vi "get_output_type.vi"(8 "error in (no error)":errorcluster, 11 "VISA Refnum in":refnum<visa-resource-name>) -> (0 "error out":errorcluster, 2 "Output type":string, 3 "VISA Refnum out":refnum<visa-resource-name>)   [LabVIEW 2018]
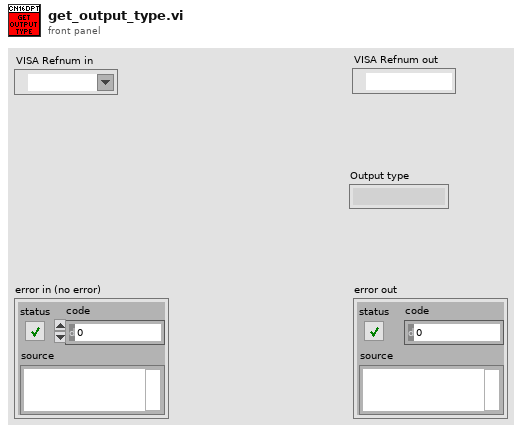
[diagram p1: front panel]
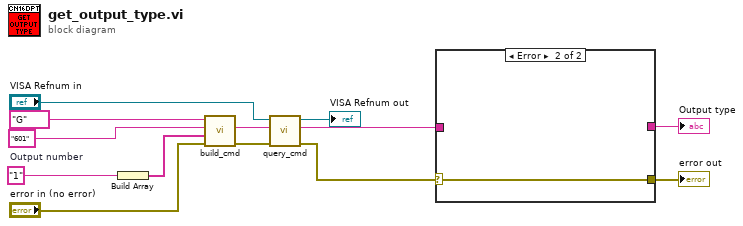
[diagram p0: block diagram]
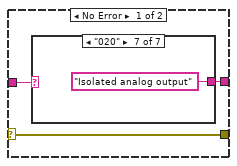
[diagram p2: hidden frame]
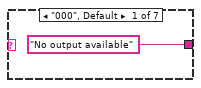
[diagram p3: hidden frame]
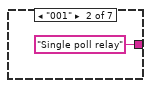
[diagram p4: hidden frame]
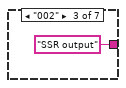
[diagram p5: hidden frame]
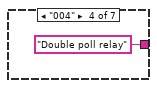
[diagram p6: hidden frame]
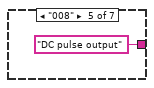
[diagram p7: hidden frame]
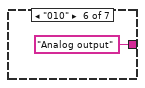
[diagram p8: hidden frame]
diagram:
  w3 = "1"  # Output number
  n1 = Build Array(w3) -> (w2:string[])
  n2 = call "build_cmd.vi"("error in (no error)"="error in (no error)", "Parameter list"=w2, "Command ID"="601", "Command class"="G") -> ("error out"=w8:errorcluster, "Command"=w7:string)  [unwired: 6 in]
  n3 = call "query_cmd.vi"("error in (no error)"=w8, "Command"=w7, "VISA resource name"="VISA Refnum in") -> ("error out"=w6:errorcluster, "Response"=w5:string, "VISA resource name out"=→"VISA Refnum out":refnum<visa-resource-name>)  [unwired: 6 in]
  n4 = case shown="Error" w6 {
    selector: w6 -> [w14 w24]
    tunnel: w5 -> [w16 _]
    tunnel: [w14 w24] -> w4
    tunnel: [w15 _] -> w1
    frame No Error {
      n5 = case shown="\"020\"" w16 {
        tunnel: ["No output available" "Single poll relay" "SSR output" "Double poll relay" "DC pulse output" "Analog output" "Isolated analog output"] -> w15
        frame "000", Default {
        }
        frame "001" {
        }
        frame "002" {
        }
        frame "004" {
        }
        frame "008" {
        }
        frame "010" {
        }
        frame "020" {
        }
      }
    }
    frame Error {
    }
  }
  "error out" <- w4
  "Output type" <- w1
